vi "Read Key (String).vi"(4 "multibyte encoding (0: None)":u16(ring) items=["None", "Shift-JIS"], 6 "read raw string? (F)":bool, 7 "section":string, 8 "error in (no error)":errorcluster, 9 "default value":string, 10 "key":string, 11 "refnum":T1) -> (0 "error out":errorcluster, 1 "value":string, 2 "found?":bool, 3 "refnum out":T1)   [LabVIEW 2009]
doc: "Reads a value associated with a key in a specified section from the configuration data identified by <B>refnum</B>. If the key does not exist, the VI returns the default value. You can use this polymorphic VI to read the following types of values from a key: Boolean, double-precision numeric, signed integer, path, string, and unsigned integer. The data type you wire to the <B>default value</B> input determines the polymorphic instance to use."
uses:
  <vilib>/Utility/config.llb/Config Data RefNum.ctl
  <vilib>/Utility/config.llb/NI_LVConfig.lvlib
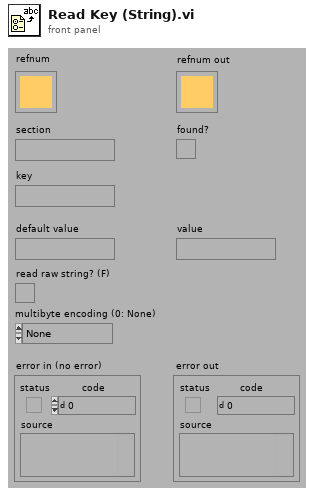
[diagram p1: front panel]
types:
  T1 = typedef "NI_LVConfig.lvlib/Config Data RefNum.ctl" = refnum<k1>
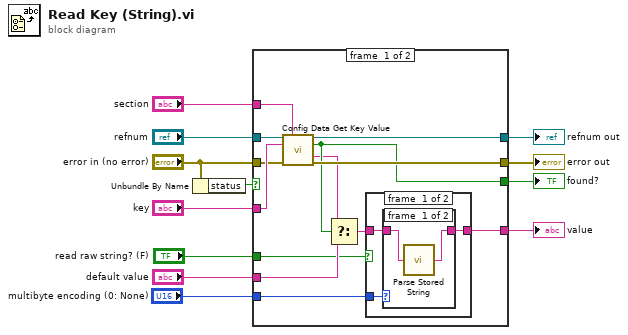
[diagram p0: block diagram]
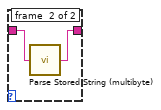
[diagram p2: hidden frame]
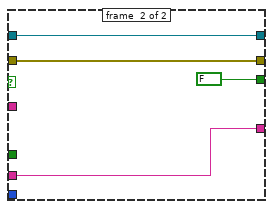
[diagram p4: hidden frame]
diagram:
  n1 = Unbundle By Name("error in (no error)") -> ("status"=w4:bool)
  n2 = case shown="False" w4 {
    tunnel: [w23 w36] -> w12
    tunnel: [w22 w37] -> w11
    tunnel: "refnum" -> [w20 w36]
    tunnel: "error in (no error)" -> [w21 w37]
    tunnel: "section" -> [w25 _]
    tunnel: "key" -> [w24 _]
    tunnel: [w19 FALSE ("section exists?")] -> w7
    tunnel: [w14 w35] -> w6
    tunnel: "default value" -> [w17 w35]
    tunnel: "read raw string? (F)" -> [w15 _]
    tunnel: "multibyte encoding (0: None)" -> [w13 _]
    frame #0 {
      n3 = call "Config Data Get Key Value.vi"("config data"=w20, "section"=w25, "key"=w24, "error in (no error)"=w21) -> ("config data out"=w23:T1, "key exists?"=w19:bool, "key value"=w18:string, "error out"=w22:errorcluster)  [unwired: 6 in, 2 out]
      n4 = Select(t=w18, s=w19, f=w17) -> (s? t:f=w16:string)
      n5 = case shown="False" w15 {
        tunnel: [w28 w33] -> w14
        tunnel: w16 -> [w27 w33]
        tunnel: w13 -> [w26 _]
        frame #0 {
          n6 = case shown="1" w26 {
            tunnel: [w30 w31] -> w28
            tunnel: w27 -> [w29 w32]
            frame #0 {
              n7 = call "Parse Stored String.vi"("stored string"=w29) -> ("parsed string"=w30:string)
            }
            frame #1 {
              n8 = call "Parse Stored String (multibyte).vi"("stored string"=w32) -> ("parsed string"=w31:string)
            }
          }
        }
        frame #1 {
        }
      }
    }
    frame #1 {
    }
  }
  "error out" <- w11
  "refnum out" <- w12
  "value" <- w6
  "found?" <- w7
